vi "gpib_build_visa_resource_name.vi"(7 "test mode":T1(ring), 8 "error in (no error)":errorcluster, 10 "GPIB settings":T2) -> (0 "error out":errorcluster, 1 "VISA Resource name 2":refnum<visa-resource-name>, 3 "VISA Resource name 1":refnum<visa-resource-name>)   [LabVIEW 2015]
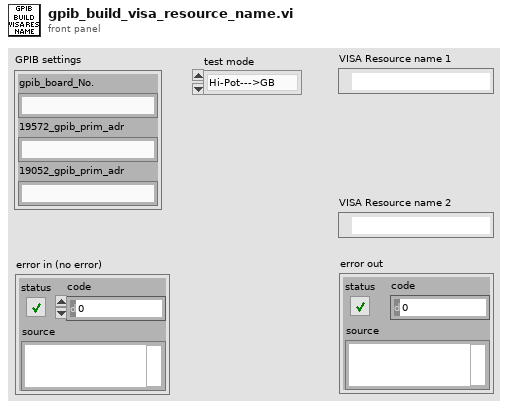
[diagram p1: front panel]
types:
  T1 = enum16{"Hi-Pot--->GB", "GB--->Hi-Pot", "Hi-Pot only", "GB only"}
  T2 = cluster{"gpib_board_No.":string, "19572_gpib_prim_adr":string, "19052_gpib_prim_adr":string}
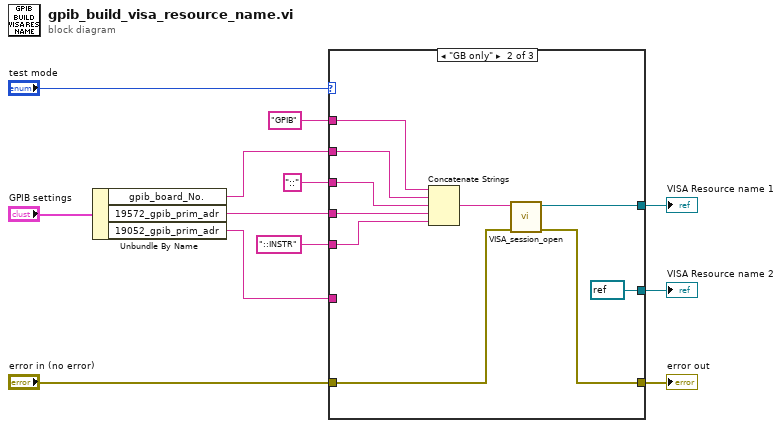
[diagram p0: block diagram]
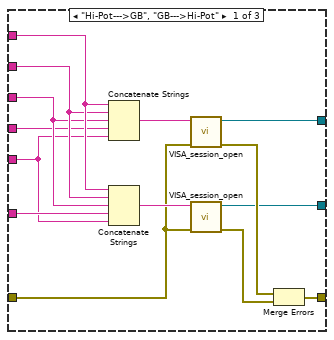
[diagram p2: hidden frame]
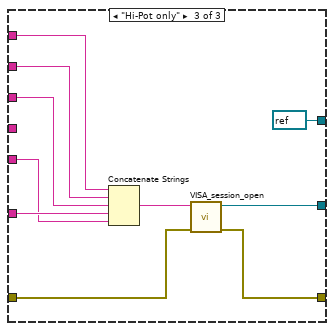
[diagram p3: hidden frame]
diagram:
  n1 = Unbundle By Name("GPIB settings") -> ("gpib_board_No."=w4:string, "19572_gpib_prim_adr"=w3:string, "19052_gpib_prim_adr"=w2:string)
  n2 = case shown="\"GB only\"" "test mode" {
    tunnel: w3 -> [w17 w30 _]
    tunnel: w2 -> [w16 _ w38]
    tunnel: [w25 w35 refnum<visa-resource-name> refnum ("VISA resource out 2")] -> w11
    tunnel: [w14 refnum<visa-resource-name> refnum ("VISA resource out 2") w39] -> w12
    tunnel: "error in (no error)" -> [w13 w28 w45]
    tunnel: [w21 w34 w44] -> w10
    tunnel: w4 -> [w19 w32 w43]
    tunnel: "GPIB" -> [w20 w33 w42]
    tunnel: "::" ("string") -> [w18 w31 w41]
    tunnel: "::INSTR" -> [w15 w29 w37]
    frame "Hi-Pot--->GB", "GB--->Hi-Pot" {
      n3 = Concatenate Strings(w20, w19, w18, w17, w15) -> (w26:string)
      n4 = Concatenate Strings(w20, w19, w18, w16, w15) -> (w24:string)
      n5 = call "VISA_session_open.vi"("error in (no error)"=w13, "VISA resource name"=w26) -> ("error out"=w22:errorcluster, "VISA resource name out"=w25:refnum<visa-resource-name>)  [unwired: 8 in]
      n6 = call "VISA_session_open.vi"("error in (no error)"=w13, "VISA resource name"=w24) -> ("error out"=w23:errorcluster, "VISA resource name out"=w14:refnum<visa-resource-name>)  [unwired: 8 in]
      n7 = Merge Errors(w22, w23) -> (w21:errorcluster)
    }
    frame "GB only" {
      n8 = Concatenate Strings(w33, w32, w31, w30, w29) -> (w36:string)
      n9 = call "VISA_session_open.vi"("error in (no error)"=w28, "VISA resource name"=w36) -> ("error out"=w34:errorcluster, "VISA resource name out"=w35:refnum<visa-resource-name>)  [unwired: 8 in]
    }
    frame "Hi-Pot only" {
      n10 = Concatenate Strings(w42, w43, w41, w38, w37) -> (w46:string)
      n11 = call "VISA_session_open.vi"("error in (no error)"=w45, "VISA resource name"=w46) -> ("error out"=w44:errorcluster, "VISA resource name out"=w39:refnum<visa-resource-name>)  [unwired: 8 in]
    }
  }
  "VISA Resource name 2" <- w12
  "VISA Resource name 1" <- w11
  "error out" <- w10
